vi "Untitled 2.vi"() -> ()   [LabVIEW 2017]
panel:
  out "Address 2":u32 format="%.0x"
  in  "address":string="192.168.10.10"
  in  "SMA mode":bool
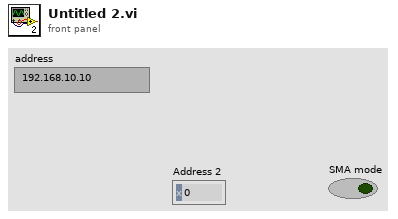
[diagram p1: front panel]
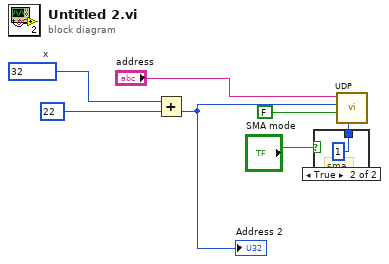
[diagram p0: block diagram]
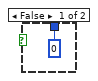
[diagram p2: hidden frame]
diagram:
  w2 = u16 32  # x
  n1 = Add(x=w2, y=u32 22 ("Address")) -> (x+y=w1:u32)
  "Address 2" <- w1
  n2 = case shown="True" "SMA mode" {
    tunnel: [u8 0 ("In") u8 1 ("In")] -> w6
    frame False {
    }
    frame True {
      # "sma"
    }
  }
  n3 = call "UDP.vi"("In"=w6, "Read (TRUE)"=FALSE, "Address"=w1, "IP address"="address") -> ()  [unwired: 5 in, 2 out]
